vi "Autoscale.vi"(8 "error in (no error)":errorcluster, 11 "Program Data":T2={"Measurements"={"Channel 0"="", "RMS 0"="", "Vp-p 0"="", "Freq 0"="", "Channel 1"="", "RMS 1"="", "Vp-p 1"="", "Freq 1"="", "Cursors"="", "C1"="", "C2"="", "dT"=""}, "C1"={"Name"="", "X"=0.0, "Y"=0.0}, "C2"={"Name"="", "X"=0.0, "Y"=0.0}, "Com"={"Connection Info"={"connection ID"=refnum, "meta data"=[]}, "Connected?"=FALSE, "IP"=""}, "Continuous?"=FALSE, "Scope Data"={"AI0"=[], "AI1"=[]}, "Wave Parameters"={"Frequency (Hz)"=0.0, "Phase offset (deg)"=0.0, "Vpeak (V)"=0.0, "Offset (V)"=0.0, "Waveform"=enum."Sine", "Channel"=enum."CH0"}, "Acquire?"=FALSE, "Measure Ref"=refnum, "CH0"={"Channel"=enum."AI 0", "Enable"=TRUE, "Volts/Div"=5, "Vertical Position (Div)"=0.0}, "CH1"={"Channel"=enum."AI 1", "Enable"=FALSE, "Volts/Div"=5, "Vertical Position (Div)"=0.0}, "CH0 Params"={"V/Div"=0.5, "Units"="V"}, "CH1 Params"={"V/Div"=0.5, "Units"="V"}, "Time"={"Time/Div"=0.0}, "dT"=0.0, "FGen"={"Offset (V)"=0.0, "Enable Sweep"=FALSE, "Start Frequency (Hz)"=0.0, "Stop Frequency (Hz)"=0.0, "Step (Hz)"=0.0, "Step Interval (ms)"=0.0, "Current Freq (Hz)"=0.0, "Run"=FALSE}} {"Time"."Time/Div" min=0.0 max=16.0 step=1.0 scale=0.0..12.0; "CH1"."Vertical Position (Div)" min=-5.0 max=5.0 step=0.1 scale=-5.0..5.0; "CH1"."Volts/Div" min=0 max=8 step=1 scale=0.0..8.0; "CH0"."Vertical Position (Div)" min=-5.0 max=5.0 step=0.1 scale=-5.0..5.0; "CH0"."Volts/Div" min=0 max=8 step=1 scale=0.0..8.0; "Wave Parameters"."Phase offset (deg)" format="%#_6p"; "Wave Parameters"."Frequency (Hz)" format="%#_6p"}) -> (0 "error out":errorcluster, 1 "CH1 Volts/Div":T1 min=0 max=8 step=1 scale=0.0..8.0, 2 "CH0 Volts/Div":T1 min=0 max=8 step=1 scale=0.0..8.0, 3 "Program Data Out":T2={"Measurements"={"Channel 0"="", "RMS 0"="", "Vp-p 0"="", "Freq 0"="", "Channel 1"="", "RMS 1"="", "Vp-p 1"="", "Freq 1"="", "Cursors"="", "C1"="", "C2"="", "dT"=""}, "C1"={"Name"="", "X"=0.0, "Y"=0.0}, "C2"={"Name"="", "X"=0.0, "Y"=0.0}, "Com"={"Connection Info"={"connection ID"=refnum, "meta data"=[]}, "Connected?"=FALSE, "IP"=""}, "Continuous?"=FALSE, "Scope Data"={"AI0"=[], "AI1"=[]}, "Wave Parameters"={"Frequency (Hz)"=0.0, "Phase offset (deg)"=0.0, "Vpeak (V)"=0.0, "Offset (V)"=0.0, "Waveform"=enum."Sine", "Channel"=enum."CH0"}, "Acquire?"=FALSE, "Measure Ref"=refnum, "CH0"={"Channel"=enum."AI 0", "Enable"=TRUE, "Volts/Div"=5, "Vertical Position (Div)"=0.0}, "CH1"={"Channel"=enum."AI 1", "Enable"=FALSE, "Volts/Div"=5, "Vertical Position (Div)"=0.0}, "CH0 Params"={"V/Div"=0.5, "Units"="V"}, "CH1 Params"={"V/Div"=0.5, "Units"="V"}, "Time"={"Time/Div"=0.0}, "dT"=0.0, "FGen"={"Offset (V)"=0.0, "Enable Sweep"=FALSE, "Start Frequency (Hz)"=0.0, "Stop Frequency (Hz)"=0.0, "Step (Hz)"=0.0, "Step Interval (ms)"=0.0, "Current Freq (Hz)"=0.0, "Run"=FALSE}} {"Time"."Time/Div" min=0.0 max=16.0 step=1.0 scale=0.0..12.0; "CH1"."Vertical Position (Div)" min=-5.0 max=5.0 step=0.1 scale=-5.0..5.0; "CH1"."Volts/Div" min=0 max=8 step=1 scale=0.0..8.0; "CH0"."Vertical Position (Div)" min=-5.0 max=5.0 step=0.1 scale=-5.0..5.0; "CH0"."Volts/Div" min=0 max=8 step=1 scale=0.0..8.0; "Wave Parameters"."Phase offset (deg)" format="%#_6p"; "Wave Parameters"."Frequency (Hz)" format="%#_6p"})   [LabVIEW 2021]
uses:
  Controls/Program Data.ctl
  Controls/Measurements.ctl
  Controls/Channel Measurement String Control.ctl
  Controls/Cursor Info.ctl
  Controls/Communication Cluster.ctl
  <vilib>/NI/STM/TCP/TCP Connection Info.ctl
  <vilib>/NI/STM/SubVIs/MetaDataElement.ctl
  Communication/Scope Data.ctl
  Program Files (x86)/National Instruments/LabVIEW 2021/ProjectTemplates/Source/myRIO/Oscilloscope/myRIO v1.1/Real-Time/Controls/Wave Parameters.ctl
  Program Files (x86)/National Instruments/LabVIEW 2021/ProjectTemplates/Source/myRIO/Oscilloscope/myRIO v1.1/Real-Time/Controls/Waveform Enum.ctl
  Program Files (x86)/National Instruments/LabVIEW 2021/ProjectTemplates/Source/myRIO/Oscilloscope/myRIO v1.1/Real-Time/Controls/Channel Selector.ctl
  Controls/Channel Settings.ctl
  Controls/Analog Input Selector.ctl
  Controls/Knob.ctl
  Controls/Vertical Position.ctl
  Controls/Channel Parameters.ctl
  Controls/Time Selector.ctl
  Controls/Time Knob.ctl
  Controls/FGen Desktop Configuration.ctl
  <vilib>/NI/STM/NI STM.lvlib
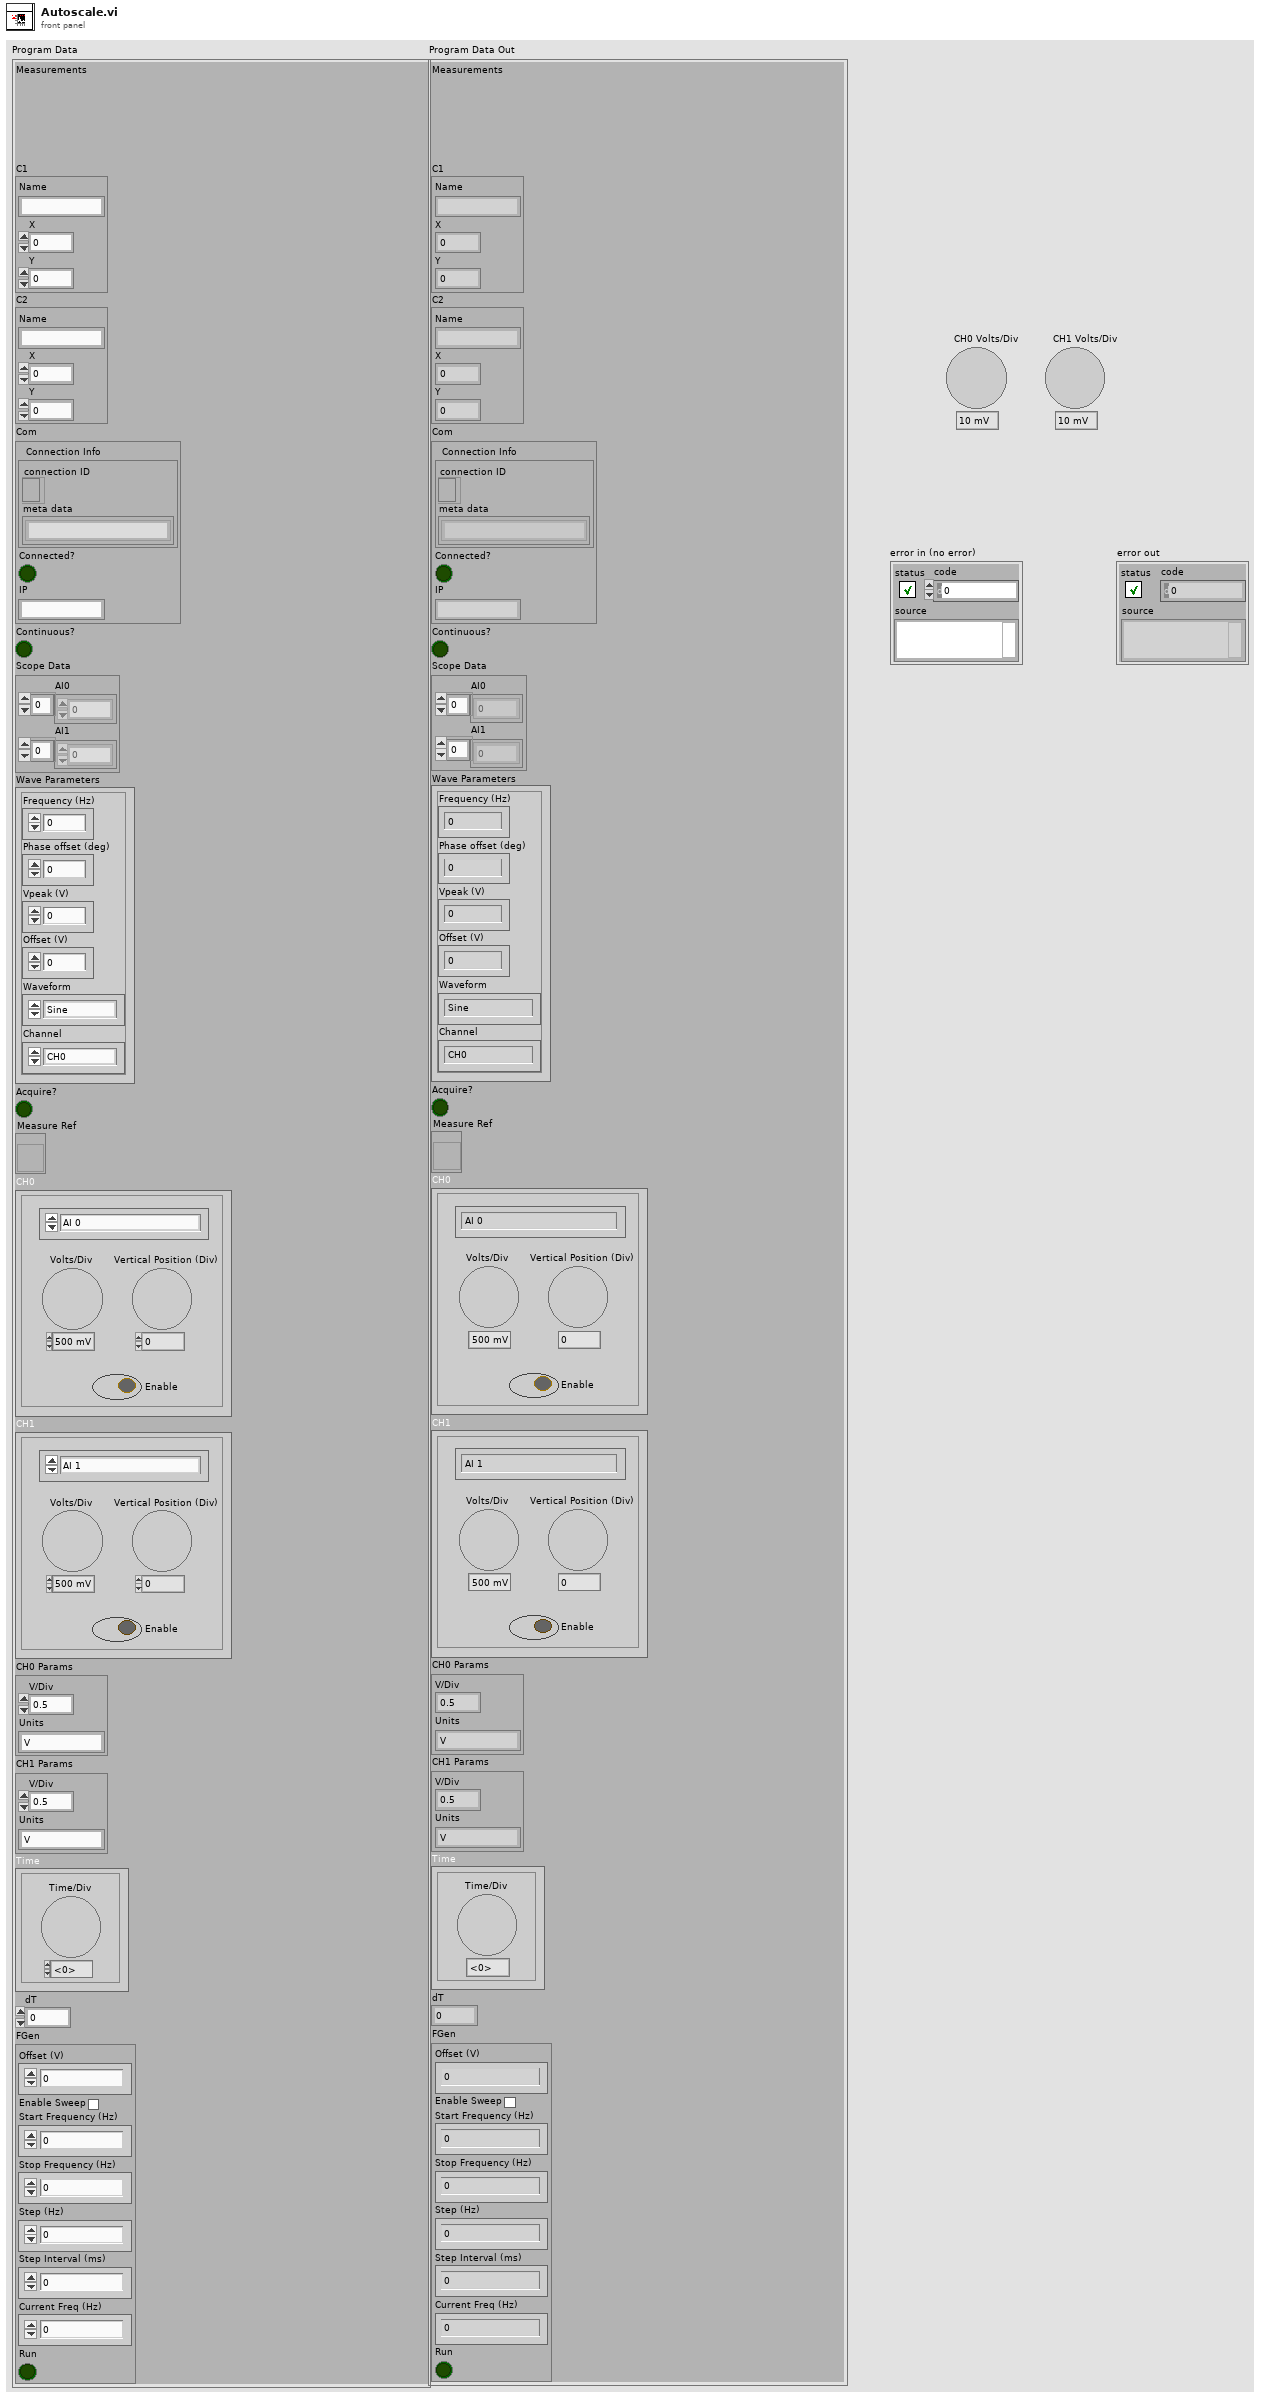
[diagram p1: front panel]
types:
  T1 = typedef "Knob.ctl" = i32
  T2 = typedef "Program Data.ctl" = cluster{"Measurements":T3, "C1":T5, "C2":T5, "Com":T6, "Continuous?":bool, "Scope Data":T9, "Wave Parameters":T10, "Acquire?":bool, "Measure Ref":refnum<vi>, "CH0":T13, "CH1":T13, "CH0 Params":T16, "CH1 Params":T16, "Time":T17, "dT":dbl, "FGen":T19}
  T3 = typedef "Measurements.ctl" = cluster{"Channel 0":T4, "RMS 0":T4, "Vp-p 0":T4, "Freq 0":T4, "Channel 1":T4, "RMS 1":T4, "Vp-p 1":T4, "Freq 1":T4, "Cursors":T4, "C1":T4, "C2":T4, "dT":T4}
  T4 = typedef "Channel Measurement String Control.ctl" = string
  T5 = typedef "Cursor Info.ctl" = cluster{"Name":string, "X":dbl, "Y":dbl}
  T6 = typedef "Communication Cluster.ctl" = cluster{"Connection Info":T7, "Connected?":bool, "IP":string}
  T7 = typedef "NI STM.lvlib/TCP Connection Info.ctl" = cluster{"connection ID":refnum<k5>, "meta data":T8[]}
  T8 = typedef "NI STM.lvlib/MetaDataElement.ctl" = string
  T9 = typedef "Scope Data.ctl" = cluster{"AI0":dbl[], "AI1":dbl[]}
  T10 = typedef "Wave Parameters.ctl" = cluster{"Frequency (Hz)":dbl, "Phase offset (deg)":dbl, "Vpeak (V)":dbl, "Offset (V)":dbl, "Waveform":T11, "Channel":T12}
  T11 = typedef "Waveform Enum.ctl" = enum16{"Sine", "Square"}
  T12 = typedef "Channel Selector.ctl" = enum16{"CH0", "CH1"}
  T13 = typedef "Channel Settings.ctl" = cluster{"Channel":T14, "Enable":bool, "Volts/Div":T1, "Vertical Position (Div)":T15}
  T14 = typedef "Analog Input Selector.ctl" = enum16{"AI 0", "AI 1"}
  T15 = typedef "Vertical Position.ctl" = dbl
  T16 = typedef "Channel Parameters.ctl" = cluster{"V/Div":dbl, "Units":string}
  T17 = typedef "Time Selector.ctl" = cluster{"Time/Div":T18}
  T18 = typedef "Time Knob.ctl" = dbl
  T19 = typedef "FGen Desktop Configuration.ctl" = cluster{"Offset (V)":dbl, "Enable Sweep":bool, "Start Frequency (Hz)":dbl, "Stop Frequency (Hz)":dbl, "Step (Hz)":dbl, "Step Interval (ms)":dbl, "Current Freq (Hz)":dbl, "Run":bool}
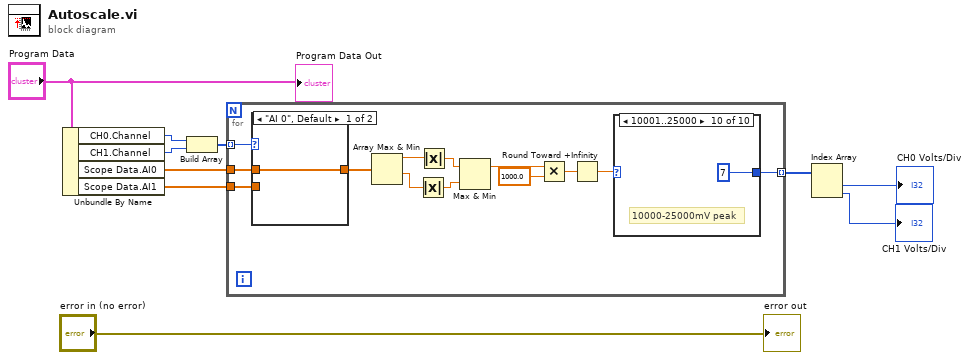
[diagram p0: block diagram]
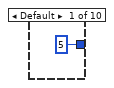
[diagram p2: hidden frame]
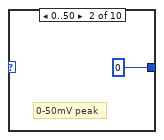
[diagram p3: hidden frame]
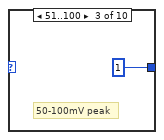
[diagram p4: hidden frame]
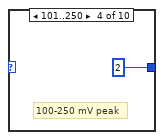
[diagram p5: hidden frame]
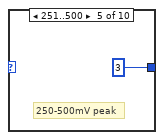
[diagram p6: hidden frame]
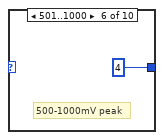
[diagram p7: hidden frame]
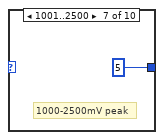
[diagram p8: hidden frame]
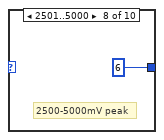
[diagram p9: hidden frame]
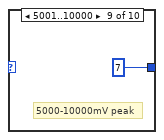
[diagram p10: hidden frame]
diagram:
  n1 = Unbundle By Name("Program Data") -> ("CH0.Channel"=w7:T14, "CH1.Channel"=w6:T14, "Scope Data.AI0"=w8:dbl[], "Scope Data.AI1"=w4:dbl[])
  n2 = Build Array(w7, w6) -> (w5:T14[])
  n3 = for {
    tunnel: w8 -> [w22]
    tunnel: w5 -> [w23] mode=indexing
    tunnel: w4 -> [w21]
    tunnel: [w11] -> w3 mode=indexing
    n4 = case shown="\"AI 0\", Default" w23 {
      tunnel: [w34 w35] -> w20
      tunnel: w22 -> [w34 _]
      tunnel: w21 -> [_ w35]
      frame "AI 0", Default {
      }
      frame "AI 1" {
      }
    }
    n5 = Array Max & Min(array=w20) -> (max value=w19:dbl, min value=w18:dbl)  [unwired: 2 out]
    n6 = Absolute Value(x=w18) -> (abs(x)=w17:dbl)
    n7 = Absolute Value(x=w19) -> (abs(x)=w16:dbl)
    n8 = Max & Min(x=w16, y=w17) -> (max(x,y)=w15:dbl)  [unwired: 1 out]
    n9 = Multiply(x=w15, y=1000.0) -> (x*y=w13:dbl)
    n10 = Round Toward +Infinity(x=w13) -> (ceil(x): smallest int >= x=w14:dbl)
    n11 = case shown="10001..25000" w14 {
      tunnel: [5 0 1 2 3 4 5 6 7 7] -> w11
      frame Default {
      }
      frame 0..50 {
        # "0-50mV peak"
      }
      frame 51..100 {
        # "50-100mV peak"
      }
      frame 101..250 {
        # "100-250 mV peak"
      }
      frame 251..500 {
        # "250-500mV peak"
      }
      frame 501..1000 {
        # "500-1000mV peak"
      }
      frame 1001..2500 {
        # "1000-2500mV peak"
      }
      frame 2501..5000 {
        # "2500-5000mV peak"
      }
      frame 5001..10000 {
        # "5000-10000mV peak"
      }
      frame 10001..25000 {
        # "10000-25000mV peak"
      }
    }
  }
  n12 = Index Array(array=w3) -> (element #1=→"CH0 Volts/Div":i32, element #2=→"CH1 Volts/Div":i32)  [unwired: 2 in]
  "Program Data Out" <- "Program Data"
  "error out" <- "error in (no error)"
